vi "linspace.vi"   [LabVIEW 2010]
uses:
  common.lvlib
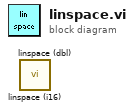
[diagram p0: block diagram]
diagram:
  n1 = call "linspace (i16).vi"() -> ()  [unwired: 11 in, 1 out]
  n2 = call "linspace (dbl).vi"() -> ()  [unwired: 11 in, 1 out]
